vi "Is At Prompt.vi"(8 "error in (no error)":errorcluster, 11 "DeployResource in":refnum<class "DeployResource.lvclass">) -> (0 "error out":errorcluster, 2 "At Prompt?":bool, 3 "DeployResource out":refnum<class "DeployResource.lvclass">, 5 "Returned Data":string)   [LabVIEW 2020, in "PicoG-Core.lvlib" / "DeployResource.lvclass"]
uses:
  DeployResource.lvclass
panel:
  # "Can remove this later.\nNow, it helps with error debug."
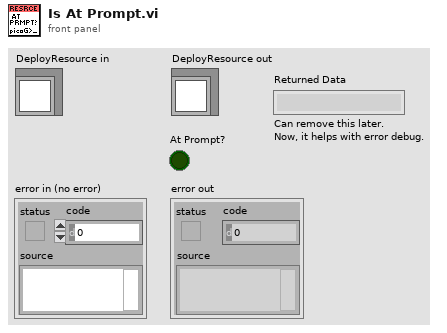
[diagram p1: front panel]
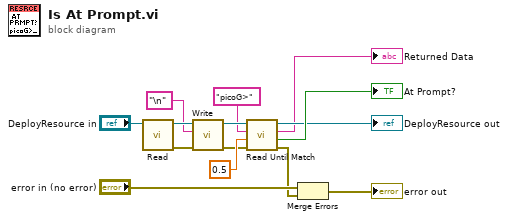
[diagram p0: block diagram]
diagram:
  n1 = call "Read.vi"("DeployResource in"="DeployResource in") -> ("error out"=w11:errorcluster, "DeployResource out"=w10:refnum<class "DeployResource.lvclass">)  [unwired: 7 in, 2 out]
  n2 = call "Write.vi"("error in (no error)"=w11, "Data"="\n", "DeployResource in"=w10) -> ("error out"=w3:errorcluster, "DeployResource out"=w8:refnum<class "DeployResource.lvclass">)  [unwired: 6 in, 1 out]
  n3 = call "Read Until Match.vi"("error in (no error)"=w3, "Timeout S (0)"=0.5, "Match String"="picoG>" ("regular expression"), "DeployResource in"=w8) -> ("error out"=w4:errorcluster, "Found?"=→"At Prompt?":bool, "Data"=→"Returned Data":string, "DeployResource out"=→"DeployResource out":refnum<class "DeployResource.lvclass">)  [unwired: 4 in]
  n4 = Merge Errors("error in (no error)", w4) -> (→"error out":errorcluster)
